vi "Methods to Tree Arr_2.vi"(7 "Action":T1, 10 "Class":string, 11 "Methods[]":T3(array[cluster])) -> (3 "Properties for Tree Out":T2(array[cluster]))   [LabVIEW 2023] (continued)
Tag", "Long name (localized)"="Tag:Delete"}, "Method Flags"={"IsDeprecated"=FALSE, "IsPrivate"=FALSE, "IsScripting"=FALSE, "IsNotInRun-Time"=TRUE}, "Divider"=FALSE}, {"Class Info"={"Unique ID string"="74", "Parent ID string"="", "Class Name (unlocalized)"="ProjectItem", "Class Name (localized)"="ProjectItem"}, "Method Info"={"Unique ID string"="35b5380f", "Data name"="Get Tag Names", "Short name (localized)"="Get Tag Names", "Long name (localized)"="Tag:Get Names"}, "Method Flags"={"IsDeprecated"=FALSE, "IsPrivate"=FALSE, "IsScripting"=FALSE, "IsNotInRun-Time"=FALSE}, "Divider"=FALSE}, {"Class Info"={"Unique ID string"="74", "Parent ID string"="", "Class Name (unlocalized)"="ProjectItem", "Class Name (localized)"="ProjectItem"}, "Method Info"={"Unique ID string"="35b53810", "Data name"="Get All Descendents", "Short name (localized)"="Get All Descendents", "Long name (localized)"="Get All Descendents"}, "Method Flags"={"IsDeprecated"=FALSE, "IsPrivate"=FALSE, "IsScripting"=FALSE, "IsNotInRun-Time"=FALSE}, "Divider"=FALSE}, {"Class Info"={"Unique ID string"="74", "Parent ID string"="", "Class Name (unlocalized)"="ProjectItem", "Class Name (localized)"="ProjectItem"}, "Method Info"={"Unique ID string"="35b53811", "Data name"="Make Item Visible in Tree", "Short name (localized)"="Make Item Visible in Tree", "Long name (localized)"="Make Item Visible in Tree"}, "Method Flags"={"IsDeprecated"=FALSE, "IsPrivate"=TRUE, "IsScripting"=FALSE, "IsNotInRun-Time"=TRUE}, "Divider"=FALSE}, {"Class Info"={"Unique ID string"="74", "Parent ID string"="", "Class Name (unlocalized)"="ProjectItem", "Class Name (localized)"="ProjectItem"}, "Method Info"={"Unique ID string"="35b53812", "Data name"="SelectItem", "Short name (localized)"="SelectItem", "Long name (localized)"="Select Item"}, "Method Flags"={"IsDeprecated"=FALSE, "IsPrivate"=TRUE, "IsScripting"=FALSE, "IsNotInRun-Time"=TRUE}, "Divider"=FALSE}, {"Class Info"={"Unique ID string"="74", "Parent ID string"="", "Class Name (unlocalized)"="ProjectItem", "Class Name (localized)"="ProjectItem"}, "Method Info"={"Unique ID string"="35b53813", "Data name"="SimulateDragSelection", "Short name (localized)"="SimulateDragSelection", "Long name (localized)"="Simulate:Drag Selection"}, "Method Flags"={"IsDeprecated"=FALSE, "IsPrivate"=TRUE, "IsScripting"=FALSE, "IsNotInRun-Time"=TRUE}, "Divider"=FALSE}, {"Class Info"={"Unique ID string"="74", "Parent ID string"="", "Class Name (unlocalized)"="ProjectItem", "Class Name (localized)"="ProjectItem"}, "Method Info"={"Unique ID string"="35b53814", "Data name"="Simulate Copy", "Short name (localized)"="Simulate Copy", "Long name (localized)"="Simulate:Copy"}, "Method Flags"={"IsDeprecated"=FALSE, "IsPrivate"=TRUE, "IsScripting"=FALSE, "IsNotInRun-Time"=TRUE}, "Divider"=FALSE}, {"Class Info"={"Unique ID string"="74", "Parent ID string"="", "Class Name (unlocalized)"="ProjectItem", "Class Name (localized)"="ProjectItem"}, "Method Info"={"Unique ID string"="35b53815", "Data name"="Simulate Paste", "Short name (localized)"="Simulate Paste", "Long name (localized)"="Simulate:Paste"}, "Method Flags"={"IsDeprecated"=FALSE, "IsPrivate"=TRUE, "IsScripting"=FALSE, "IsNotInRun-Time"=TRUE}, "Divider"=FALSE}, {"Class Info"={"Unique ID string"="74", "Parent ID string"="", "Class Name (unlocalized)"="ProjectItem", "Class Name (localized)"="ProjectItem"}, "Method Info"={"Unique ID string"="35b53816", "Data name"="Simulate Drag To VI", "Short name (localized)"="Simulate Drag To VI", "Long name (localized)"="Simulate:Drag To VI"}, "Method Flags"={"IsDeprecated"=FALSE, "IsPrivate"=TRUE, "IsScripting"=FALSE, "IsNotInRun-Time"=TRUE}, "Divider"=FALSE}, {"Class Info"={"Unique ID string"="74", "Parent ID string"="", "Class Name (unlocalized)"="ProjectItem", "Class Name (localized)"="ProjectItem"}, "Method Info"={"Unique ID string"="35b53817", "Data name"="Simulate Paste To VI", "Short name (localized)"="Simulate Paste To VI", "Long name (localized)"="Simulate:Paste To VI"}, "Method Flags"={"IsDeprecated"=FALSE, "IsPrivate"=TRUE, "IsScripting"=FALSE, "IsNotInRun-Time"=TRUE}, "Divider"=FALSE}, {"Class Info"={"Unique ID string"="74", "Parent ID string"="", "Class Name (unlocalized)"="ProjectItem", "Class Name (localized)"="ProjectItem"}, "Method Info"={"Unique ID string"="35b53818", "Data name"="Simulate Drag From Paths", "Short name (localized)"="Simulate Drag From Paths", "Long name (localized)"="Simulate:Drag From Paths"}, "Method Flags"={"IsDeprecated"=FALSE, "IsPrivate"=TRUE, "IsScripting"=FALSE, "IsNotInRun-Time"=TRUE}, "Divider"=FALSE}, {"Class Info"={"Unique ID string"="74", "Parent ID string"="", "Class Name (unlocalized)"="ProjectItem", "Class Name (localized)"="ProjectItem"}, "Method Info"={"Unique ID string"="35b53819", "Data name"="Collapse", "Short name (localized)"="Collapse", "Long name (localized)"="Collapse"}, "Method Flags"={"IsDeprecated"=FALSE, "IsPrivate"=FALSE, "IsScripting"=FALSE, "IsNotInRun-Time"=TRUE}, "Divider"=FALSE}, {"Class Info"={"Unique ID string"="74", "Parent ID string"="", "Class Name (unlocalized)"="ProjectItem", "Class Name (localized)"="ProjectItem"}, "Method Info"={"Unique ID string"="35b5381a", "Data name"="Rename", "Short name (localized)"="Rename", "Long name (localized)"="Rename"}, "Method Flags"={"IsDeprecated"=FALSE, "IsPrivate"=TRUE, "IsScripting"=FALSE, "IsNotInRun-Time"=TRUE}, "Divider"=FALSE}, {"Class Info"={"Unique ID string"="74", "Parent ID string"="", "Class Name (unlocalized)"="ProjectItem", "Class Name (localized)"="ProjectItem"}, "Method Info"={"Unique ID string"="35b5381b", "Data name"="New from Template", "Short name (localized)"="New from Template", "Long name (localized)"="New from Template"}, "Method Flags"={"IsDeprecated"=FALSE, "IsPrivate"=TRUE, "IsScripting"=FALSE, "IsNotInRun-Time"=TRUE}, "Divider"=FALSE}, {"Class Info"={"Unique ID string"="74", "Parent ID string"="", "Class Name (unlocalized)"="ProjectItem", "Class Name (localized)"="ProjectItem"}, "Method Info"={"Unique ID string"="35b5381c", "Data name"="Suppress Project Dlgs", "Short name (localized)"="Suppress Project Dlgs", "Long name (localized)"="Suppress Project Dialogs"}, "Method Flags"={"IsDeprecated"=FALSE, "IsPrivate"=TRUE, "IsScripting"=FALSE, "IsNotInRun-Time"=TRUE}, "Divider"=FALSE}, {"Class Info"={"Unique ID string"="74", "Parent ID string"="", "Class Name (unlocalized)"="ProjectItem", "Class Name (localized)"="ProjectItem"}, "Method Info"={"Unique ID string"="35b5381d", "Data name"="SimulateNotify", "Short name (localized)"="SimulateNotify", "Long name (localized)"="Simulate:Notify"}, "Method Flags"={"IsDeprecated"=FALSE, "IsPrivate"=TRUE, "IsScripting"=FALSE, "IsNotInRun-Time"=TRUE}, "Divider"=FALSE}, {"Class Info"={"Unique ID string"="74", "Parent ID string"="", "Class Name (unlocalized)"="ProjectItem", "Class Name (localized)"="ProjectItem"}, "Method Info"={"Unique ID string"="35b5381e", "Data name"="SCC Get Info", "Short name (localized)"="SCC Get Info", "Long name (localized)"="SCC Get Info"}, "Method Flags"={"IsDeprecated"=FALSE, "IsPrivate"=TRUE, "IsScripting"=FALSE, "IsNotInRun-Time"=TRUE}, "Divider"=FALSE}, {"Class Info"={"Unique ID string"="74", "Parent ID string"="", "Class Name (unlocalized)"="ProjectItem", "Class Name (localized)"="ProjectItem"}, "Method Info"={"Unique ID string"="35b5381f", "Data name"="Query Behavior", "Short name (localized)"="Query Behavior", "Long name (localized)"="Query Behavior"}, "Method Flags"={"IsDeprecated"=FALSE, "IsPrivate"=TRUE, "IsScripting"=FALSE, "IsNotInRun-Time"=TRUE}, "Divider"=FALSE}, {"Class Info"={"Unique ID string"="74", "Parent ID string"="", "Class Name (unlocalized)"="ProjectItem", "Class Name (localized)"="ProjectItem"}, "Method Info"={"Unique ID string"="35b53820", "Data name"="Move", "Short name (localized)"="Move", "Long name (localized)"="Move"}, "Method Flags"={"IsDeprecated"=FALSE, "IsPrivate"=TRUE, "IsScripting"=FALSE, "IsNotInRun-Time"=TRUE}, "Divider"=FALSE}, {"Class Info"={"Unique ID string"="74", "Parent ID string"="", "Class Name (unlocalized)"="ProjectItem", "Class Name (localized)"="ProjectItem"}, "Method Info"={"Unique ID string"="35b53821", "Data name"="Delete Privately", "Short name (localized)"="Delete Privately", "Long name (localized)"="Delete Privately (tell no outsiders)"}, "Method Flags"={"IsDeprecated"=FALSE, "IsPrivate"=TRUE, "IsScripting"=FALSE, "IsNotInRun-Time"=TRUE}, "Divider"=FALSE}, {"Class Info"={"Unique ID string"="74", "Parent ID string"="", "Class Name (unlocalized)"="ProjectItem", "Class Name (localized)"="ProjectItem"}, "Method Info"={"Unique ID string"="35b53822", "Data name"="Get XML Tag", "Short name (localized)"="Get XML Tag", "Long name (localized)"="Tag:Get XML Tag"}, "Method Flags"={"IsDeprecated"=FALSE, "IsPrivate"=FALSE, "IsScripting"=FALSE, "IsNotInRun-Time"=FALSE}, "Divider"=FALSE}, {"Class Info"={"Unique ID string"="74", "Parent ID string"="", "Class Name (unlocalized)"="ProjectItem", "Class Name (localized)"="ProjectItem"}, "Method Info"={"Unique ID string"="35b53823", "Data name"="Set XML Tag", "Short name (localized)"="Set XML Tag", "Long name (localized)"="Tag:Set XML Tag"}, "Method Flags"={"IsDeprecated"=FALSE, "IsPrivate"=FALSE, "IsScripting"=FALSE, "IsNotInRun-Time"=TRUE}, "Divider"=FALSE}, {"Class Info"={"Unique ID string"="74", "Parent ID string"="", "Class Name (unlocalized)"="ProjectItem", "Class Name (localized)"="ProjectItem"}, "Method Info"={"Unique ID string"="35b53824", "Data name"="AddItemFromMemory", "Short name (localized)"="AddItemFromMemory", "Long name (localized)"="Add Item From Memory"}, "Method Flags"={"IsDeprecated"=FALSE, "IsPrivate"=FALSE, "IsScripting"=FALSE, "IsNotInRun-Time"=TRUE}, "Divider"=FALSE}, {"Class Info"={"Unique ID string"="74", "Parent ID string"="", "Class Name (unlocalized)"="ProjectItem", "Class Name (localized)"="ProjectItem"}, "Method Info"={"Unique ID string"="35b53825", "Data name"="NotifyItemChanged", "Short name (localized)"="NotifyItemChanged", "Long name (localized)"="Notify Item Changed"}, "Method Flags"={"IsDeprecated"=FALSE, "IsPrivate"=TRUE, "IsScripting"=FALSE, "IsNotInRun-Time"=TRUE}, "Divider"=FALSE}, {"Class Info"={"Unique ID string"="74", "Parent ID string"="", "Class Name (unlocalized)"="ProjectItem", "Class Name (localized)"="ProjectItem"}, "Method Info"={"Unique ID string"="35b53826", "Data name"="Expand", "Short name (localized)"="Expand", "Long name (localized)"="Expand"}, "Method Flags"={"IsDeprecated"=FALSE, "IsPrivate"=FALSE, "IsScripting"=FALSE, "IsNotInRun-Time"=TRUE}, "Divider"=FALSE}, {"Class Info"={"Unique ID string"="74", "Parent ID string"="", "Class Name (unlocalized)"="ProjectItem", "Class Name (localized)"="ProjectItem"}, "Method Info"={"Unique ID string"="35b53827", "Data name"="Arrange By", "Short name (localized)"="Arrange By", "Long name (localized)"="Arrange By"}, "Method Flags"={"IsDeprecated"=FALSE, "IsPrivate"=TRUE, "IsScripting"=FALSE, "IsNotInRun-Time"=TRUE}, "Divider"=FALSE}, {"Class Info"={"Unique ID string"="74", "Parent ID string"="", "Class Name (unlocalized)"="ProjectItem", "Class Name (localized)"="ProjectItem"}, "Method Info"={"Unique ID string"="35b53828", "Data name"="SetUrl", "Short name (localized)"="SetUrl", "Long name (localized)"="Set Url"}, "Method Flags"={"IsDeprecated"=FALSE, "IsPrivate"=TRUE, "IsScripting"=FALSE, "IsNotInRun-Time"=TRUE}, "Divider"=FALSE}, {"Class Info"={"Unique ID string"="74", "Parent ID string"="", "Class Name (unlocalized)"="ProjectItem", "Class Name (localized)"="ProjectItem"}, "Method Info"={"Unique ID string"="35b53829", "Data name"="Get All Descendents2", "Short name (localized)"="Get All Descendents2", "Long name (localized)"="Get All Descendents2"}, "Method Flags"={"IsDeprecated"=FALSE, "IsPrivate"=TRUE, "IsScripting"=FALSE, "IsNotInRun-Time"=FALSE}, "Divider"=FALSE}, {"Class Info"={"Unique ID string"="74", "Parent ID string"="", "Class Name (unlocalized)"="ProjectItem", "Class Name (localized)"="ProjectItem"}, "Method Info"={"Unique ID string"="35b5382a", "Data name"="GetFindResults", "Short name (localized)"="GetFindResults", "Long name (localized)"="GetFindResults"}, "Method Flags"={"IsDeprecated"=FALSE, "IsPrivate"=TRUE, "IsScripting"=FALSE, "IsNotInRun-Time"=FALSE}, "Divider"=FALSE}, {"Class Info"={"Unique ID string"="74", "Parent ID string"="", "Class Name (unlocalized)"="ProjectItem", "Class Name (localized)"="ProjectItem"}, "Method Info"={"Unique ID string"="35b5382b", "Data name"="Convert to Auto-populating Folder", "Short name (localized)"="Convert to Auto-populating Folder", "Long name (localized)"="Convert to Auto-populating Folder"}, "Method Flags"={"IsDeprecated"=FALSE, "IsPrivate"=FALSE, "IsScripting"=FALSE, "IsNotInRun-Time"=TRUE}, "Divider"=FALSE}, {"Class Info"={"Unique ID string"="74", "Parent ID string"="", "Class Name (unlocalized)"="ProjectItem", "Class Name (localized)"="ProjectItem"}, "Method Info"={"Unique ID string"="35b5382c", "Data name"="Stop Auto-populating", "Short name (localized)"="Stop Auto-populating", "Long name (localized)"="Stop Auto-populating"}, "Method Flags"={"IsDeprecated"=FALSE, "IsPrivate"=FALSE, "IsScripting"=FALSE, "IsNotInRun-Time"=TRUE}, "Divider"=FALSE}, {"Class Info"={"Unique ID string"="74", "Parent ID string"="", "Class Name (unlocalized)"="ProjectItem", "Class Name (localized)"="ProjectItem"}, "Method Info"={"Unique ID string"="35b5382d", "Data name"="Delete On Disk", "Short name (localized)"="Delete On Disk", "Long name (localized)"="Delete On Disk"}, "Method Flags"={"IsDeprecated"=FALSE, "IsPrivate"=TRUE, "IsScripting"=FALSE, "IsNotInRun-Time"=FALSE}, "Divider"=FALSE}, {"Class Info"={"Unique ID string"="74", "Parent ID string"="", "Class Name (unlocalized)"="ProjectItem", "Class Name (localized)"="ProjectItem"}, "Method Info"={"Unique ID string"="35b5382e", "Data name"="ListOfReferProjItems", "Short name (localized)"="ListOfReferProjItems", "Long name (localized)"="List of Refer ProjectItems"}, "Method Flags"={"IsDeprecated"=FALSE, "IsPrivate"=TRUE, "IsScripting"=FALSE, "IsNotInRun-Time"=FALSE}, "Divider"=FALSE}, {"Class Info"={"Unique ID string"="74", "Parent ID string"="", "Class Name (unlocalized)"="ProjectItem", "Class Name (localized)"="ProjectItem"}, "Method Info"={"Unique ID string"="35b5382f", "Data name"="ReplaceWithProjItem", "Short name (localized)"="ReplaceWithProjItem", "Long name (localized)"="Replace With Item in Project"}, "Method Flags"={"IsDeprecated"=FALSE, "IsPrivate"=TRUE, "IsScripting"=FALSE, "IsNotInRun-Time"=FALSE}, "Divider"=FALSE}, {"Class Info"={"Unique ID string"="74", "Parent ID string"="", "Class Name (unlocalized)"="ProjectItem", "Class Name (localized)"="ProjectItem"}, "Method Info"={"Unique ID string"="35b53830", "Data name"="Choose Substitute", "Short name (localized)"="Choose Substitute", "Long name (localized)"="Choose Substitute"}, "Method Flags"={"IsDeprecated"=FALSE, "IsPrivate"=TRUE, "IsScripting"=FALSE, "IsNotInRun-Time"=FALSE}, "Divider"=FALSE}, {"Class Info"={"Unique ID string"="74", "Parent ID string"="", "Class Name (unlocalized)"="ProjectItem", "Class Name (localized)"="ProjectItem"}, "Method Info"={"Unique ID string"="35b53831", "Data name"="AddMultipleItems", "Short name (localized)"="AddMultipleItems", "Long name (localized)"="AddMultipleItems"}, "Method Flags"={"IsDeprecated"=FALSE, "IsPrivate"=TRUE, "IsScripting"=FALSE, "IsNotInRun-Time"=FALSE}, "Divider"=FALSE}, {"Class Info"={"Unique ID string"="74", "Parent ID string"="", "Class Name (unlocalized)"="ProjectItem", "Class Name (localized)"="ProjectItem"}, "Method Info"={"Unique ID string"="35b53832", "Data name"="ForceDelete", "Short name (localized)"="ForceDelete", "Long name (localized)"="ForceDelete"}, "Method Flags"={"IsDeprecated"=FALSE, "IsPrivate"=TRUE, "IsScripting"=FALSE, "IsNotInRun-Time"=FALSE}, "Divider"=FALSE}, {"Class Info"={"Unique ID string"="74", "Parent ID string"="", "Class Name (unlocalized)"="ProjectItem", "Class Name (localized)"="ProjectItem"}, "Method Info"={"Unique ID string"="35b53833", "Data name"="Bounds", "Short name (localized)"="Bounds", "Long name (localized)"="Bounds"}, "Method Flags"={"IsDeprecated"=FALSE, "IsPrivate"=TRUE, "IsScripting"=FALSE, "IsNotInRun-Time"=FALSE}, "Divider"=FALSE}, {"Class Info"={"Unique ID string"="74", "Parent ID string"="", "Class Name (unlocalized)"="ProjectItem", "Class Name (localized)"="ProjectItem"}, "Method Info"={"Unique ID string"="35b53834", "Data name"="GetVariableURLs", "Short name (localized)"="GetVariableURLs", "Long name (localized)"="Get Variable URLs"}, "Method Flags"={"IsDeprecated"=FALSE, "IsPrivate"=TRUE, "IsScripting"=FALSE, "IsNotInRun-Time"=TRUE}, "Divider"=FALSE}, {"Class Info"={"Unique ID string"="74", "Parent ID string"="", "Class Name (unlocalized)"="ProjectItem", "Class Name (localized)"="ProjectItem"}, "Method Info"={"Unique ID string"="35b53835", "Data name"="AddItemFromMemoryPrivately", "Short name (localized)"="AddItemFromMemoryPrivately", "Long name (localized)"="Add Item From Memory Privately"}, "Method Flags"={"IsDeprecated"=FALSE, "IsPrivate"=TRUE, "IsScripting"=FALSE, "IsNotInRun-Time"=TRUE}, "Divider"=FALSE}, {"Class Info"={"Unique ID string"="74", "Parent ID string"="", "Class Name (unlocalized)"="ProjectItem", "Class Name (localized)"="ProjectItem"}, "Method Info"={"Unique ID string"="35b53836", "Data name"="Get Library Access Scope", "Short name (localized)"="Get Library Access Scope", "Long name (localized)"="Get Library Access Scope"}, "Method Flags"={"IsDeprecated"=FALSE, "IsPrivate"=TRUE, "IsScripting"=FALSE, "IsNotInRun-Time"=TRUE}, "Divider"=FALSE}, {"Class Info"={"Unique ID string"="74", "Parent ID string"="", "Class Name (unlocalized)"="ProjectItem", "Class Name (localized)"="ProjectItem"}, "Method Info"={"Unique ID string"="35b53837", "Data name"="Replace Item With", "Short name (localized)"="Replace Item With", "Long name (localized)"="Replace Item With"}, "Method Flags"={"IsDeprecated"=FALSE, "IsPrivate"=FALSE, "IsScripting"=FALSE, "IsNotInRun-Time"=TRUE}, "Divider"=FALSE}, {"Class Info"={"Unique ID string"="75", "Parent ID string"="36", "Class Name (unlocalized)"="Pane", "Class Name (localized)"="Pane"}, "Method Info"={"Unique ID string"="64afa400", "Data name"="MakeSpace", "Short name (localized)"="MakeSpace", "Long name (localized)"="Make Space"}, "Method Flags"={"IsDeprecated"=FALSE, "IsPrivate"=FALSE, "IsScripting"=TRUE, "IsNotInRun-Time"=TRUE}, "Divider"=FALSE}, {"Class Info"={"Unique ID string"="75", "Parent ID string"="36", "Class Name (unlocalized)"="Pane", "Class Name (localized)"="Pane"}, "Method Info"={"Unique ID string"="64afa402", "Data name"="Select All", "Short name (localized)"="Select All", "Long name (localized)"="Select All"}, "Method Flags"={"IsDeprecated"=FALSE, "IsPrivate"=FALSE, "IsScripting"=TRUE, "IsNotInRun-Time"=TRUE}, "Divider"=FALSE}, {"Class Info"={"Unique ID string"="75", "Parent ID string"="36", "Class Name (unlocalized)"="Pane", "Class Name (localized)"="Pane"}, "Method Info"={"Unique ID string"="64afa403", "Data name"="Paste Selection", "Short name (localized)"="Paste Selection", "Long name (localized)"="Paste Selection"}, "Method Flags"={"IsDeprecated"=FALSE, "IsPrivate"=FALSE, "IsScripting"=TRUE, "IsNotInRun-Time"=TRUE}, "Divider"=FALSE}, {"Class Info"={"Unique ID string"="75", "Parent ID string"="36", "Class Name (unlocalized)"="Pane", "Class Name (localized)"="Pane"}, "Method Info"={"Unique ID string"="64afa404", "Data name"="Group Objects", "Short name (localized)"="Group Objects", "Long name (localized)"="Group Objects"}, "Method Flags"={"IsDeprecated"=FALSE, "IsPrivate"=FALSE, "IsScripting"=TRUE, "IsNotInRun-Time"=TRUE}, "Divider"=FALSE}, {"Class Info"={"Unique ID string"="75", "Parent ID string"="36", "Class Name (unlocalized)"="Pane", "Class Name (localized)"="Pane"}, "Method Info"={"Unique ID string"="64afa405", "Data name"="Lock Objects", "Short name (localized)"="Lock Objects", "Long name (localized)"="Lock Objects"}, "Method Flags"={"IsDeprecated"=FALSE, "IsPrivate"=FALSE, "IsScripting"=TRUE, "IsNotInRun-Time"=TRUE}, "Divider"=FALSE}, {"Class Info"={"Unique ID string"="75", "Parent ID string"="36", "Class Name (unlocalized)"="Pane", "Class Name (localized)"="Pane"}, "Method Info"={"Unique ID string"="64afa406", "Data name"="Ungroup Objects", "Short name (localized)"="Ungroup Objects", "Long name (localized)"="Ungroup Objects"}, "Method Flags"={"IsDeprecated"=FALSE, "IsPrivate"=FALSE, "IsScripting"=TRUE, "IsNotInRun-Time"=TRUE}, "Divider"=FALSE}, {"Class Info"={"Unique ID string"="75", "Parent ID string"="36", "Class Name (unlocalized)"="Pane", "Class Name (localized)"="Pane"}, "Method Info"={"Unique ID string"="64afa407", "Data name"="Unlock Objects", "Short name (localized)"="Unlock Objects", "Long name (localized)"="Unlock Objects"}, "Method Flags"={"IsDeprecated"=FALSE, "IsPrivate"=FALSE, "IsScripting"=TRUE, "IsNotInRun-Time"=TRUE}, "Divider"=FALSE}, {"Class Info"={"Unique ID string"="75", "Parent ID string"="36", "Class Name (unlocalized)"="Pane", "Class Name (localized)"="Pane"}, "Method Info"={"Unique ID string"="64afa408", "Data name"="Set Scaling", "Short name (localized)"="Set Scaling", "Long name (localized)"="Set Scaling Mode"}, "Method Flags"={"IsDeprecated"=FALSE, "IsPrivate"=FALSE, "IsScripting"=FALSE, "IsNotInRun-Time"=FALSE}, "Divider"=FALSE}, {"Class Info"={"Unique ID string"="75", "Parent ID string"="36", "Class Name (unlocalized)"="Pane", "Class Name (localized)"="Pane"}, "Method Info"={"Unique ID string"="64afa409", "Data name"="Get Scaling", "Short name (localized)"="Get Scaling", "Long name (localized)"="Get Scaling Mode"}, "Method Flags"={"IsDeprecated"=FALSE, "IsPrivate"=FALSE, "IsScripting"=FALSE, "IsNotInRun-Time"=FALSE}, "Divider"=FALSE}, {"Class Info"={"Unique ID string"="75", "Parent ID string"="36", "Class Name (unlocalized)"="Pane", "Class Name (localized)"="Pane"}, "Method Info"={"Unique ID string"="64afa40a", "Data name"="CvtPaneToPanelCoords", "Short name (localized)"="CvtPaneToPanelCoords", "Long name (localized)"="Convert Pane To Panel Coordinates"}, "Method Flags"={"IsDeprecated"=FALSE, "IsPrivate"=FALSE, "IsScripting"=FALSE, "IsNotInRun-Time"=FALSE}, "Divider"=FALSE}, {"Class Info"={"Unique ID string"="75", "Parent ID string"="36", "Class Name (unlocalized)"="Pane", "Class Name (localized)"="Pane"}, "Method Info"={"Unique ID string"="64afa40b", "Data name"="CvtPanelToPaneCoords", "Short name (localized)"="CvtPanelToPaneCoords", "Long name (localized)"="Convert Panel To Pane Coordinates"}, "Method Flags"={"IsDeprecated"=FALSE, "IsPrivate"=FALSE, "IsScripting"=FALSE, "IsNotInRun-Time"=FALSE}, "Divider"=FALSE}, {"Class Info"={"Unique ID string"="80", "Parent ID string"="74", "Class Name (unlocalized)"="Library", "Class Name (localized)"="Library"}, "Method Info"={"Unique ID string"="4d10e400", "Data name"="Set Source Scope", "Short name (localized)"="Set Source Scope", "Long name (localized)"="Source Scope:Set"}, "Method Flags"={"IsDeprecated"=FALSE, "IsPrivate"=FALSE, "IsScripting"=FALSE, "IsNotInRun-Time"=TRUE}, "Divider"=FALSE}, {"Class Info"={"Unique ID string"="80", "Parent ID string"="74", "Class Name (unlocalized)"="Library", "Class Name (localized)"="Library"}, "Method Info"={"Unique ID string"="4d10e401", "Data name"="Get Source Scope", "Short name (localized)"="Get Source Scope", "Long name (localized)"="Source Scope:Get"}, "Method Flags"={"IsDeprecated"=FALSE, "IsPrivate"=FALSE, "IsScripting"=FALSE, "IsNotInRun-Time"=FALSE}, "Divider"=FALSE}, {"Class Info"={"Unique ID string"="80", "Parent ID string"="74", "Class Name (unlocalized)"="Library", "Class Name (localized)"="Library"}, "Method Info"={"Unique ID string"="4d10e402", "Data name"="Set Lock State", "Short name (localized)"="Set Lock State", "Long name (localized)"="Lock State:Set"}, "Method Flags"={"IsDeprecated"=FALSE, "IsPrivate"=FALSE, "IsScripting"=FALSE, "IsNotInRun-Time"=TRUE}, "Divider"=FALSE}, {"Class Info"={"Unique ID string"="80", "Parent ID string"="74", "Class Name (unlocalized)"="Library", "Class Name (localized)"="Library"}, "Method Info"={"Unique ID string"="4d10e403", "Data name"="Get Lock State", "Short name (localized)"="Get Lock State", "Long name (localized)"="Lock State:Get"}, "Method Flags"={"IsDeprecated"=FALSE, "IsPrivate"=FALSE, "IsScripting"=FALSE, "IsNotInRun-Time"=FALSE}, "Divider"=FALSE}, {"Class Info"={"Unique ID string"="80", "Parent ID string"="74", "Class Name (unlocalized)"="Library", "Class Name (localized)"="Library"}, "Method Info"={"Unique ID string"="4d10e404", "Data name"="Get Lib Tag", "Short name (localized)"="Get Lib Tag", "Long name (localized)"="Library Tag:Get"}, "Method Flags"={"IsDeprecated"=FALSE, "IsPrivate"=FALSE, "IsScripting"=FALSE, "IsNotInRun-Time"=FALSE}, "Divider"=FALSE}, {"Class Info"={"Unique ID string"="80", "Parent ID string"="74", "Class Name (unlocalized)"="Library", "Class Name (localized)"="Library"}, "Method Info"={"Unique ID string"="4d10e405", "Data name"="Set Lib Tag", "Short name (localized)"="Set Lib Tag", "Long name (localized)"="Library Tag:Set"}, "Method Flags"={"IsDeprecated"=FALSE, "IsPrivate"=FALSE, "IsScripting"=FALSE, "IsNotInRun-Time"=TRUE}, "Divider"=FALSE}, {"Class Info"={"Unique ID string"="80", "Parent ID string"="74", "Class Name (unlocalized)"="Library", "Class Name (localized)"="Library"}, "Method Info"={"Unique ID string"="4d10e406", "Data name"="Delete Lib Tag", "Short name (localized)"="Delete Lib Tag", "Long name (localized)"="Library Tag:Delete"}, "Method Flags"={"IsDeprecated"=FALSE, "IsPrivate"=FALSE, "IsScripting"=FALSE, "IsNotInRun-Time"=TRUE}, "Divider"=FALSE}, {"Class Info"={"Unique ID string"="80", "Parent ID string"="74", "Class Name (unlocalized)"="Library", "Class Name (localized)"="Library"}, "Method Info"={"Unique ID string"="4d10e407", "Data name"="Get Lib Tag Names", "Short name (localized)"="Get Lib Tag Names", "Long name (localized)"="Library Tag:Get Names"}, "Method Flags"={"IsDeprecated"=FALSE, "IsPrivate"=FALSE, "IsScripting"=FALSE, "IsNotInRun-Time"=FALSE}, "Divider"=FALSE}, {"Class Info"={"Unique ID string"="80", "Parent ID string"="74", "Class Name (unlocalized)"="Library", "Class Name (localized)"="Library"}, "Method Info"={"Unique ID string"="4d10e408", "Data name"="Save", "Short name (localized)"="Save", "Long name (localized)"="Save:Library"}, "Method Flags"={"IsDeprecated"=FALSE, "IsPrivate"=FALSE, "IsScripting"=FALSE, "IsNotInRun-Time"=TRUE}, "Divider"=FALSE}, {"Class Info"={"Unique ID string"="80", "Parent ID string"="74", "Class Name (unlocalized)"="Library", "Class Name (localized)"="Library"}, "Method Info"={"Unique ID string"="4d10e409", "Data name"="Get Icon", "Short name (localized)"="Get Icon", "Long name (localized)"="Icon:Get"}, "Method Flags"={"IsDeprecated"=FALSE, "IsPrivate"=FALSE, "IsScripting"=FALSE, "IsNotInRun-Time"=FALSE}, "Divider"=FALSE}, {"Class Info"={"Unique ID string"="80", "Parent ID string"="74", "Class Name (unlocalized)"="Library", "Class Name (localized)"="Library"}, "Method Info"={"Unique ID string"="4d10e40a", "Data name"="Set Icon", "Short name (localized)"="Set Icon", "Long name (localized)"="Icon:Set"}, "Method Flags"={"IsDeprecated"=FALSE, "IsPrivate"=FALSE, "IsScripting"=FALSE, "IsNotInRun-Time"=TRUE}, "Divider"=FALSE}, {"Class Info"={"Unique ID string"="80", "Parent ID string"="74", "Class Name (unlocalized)"="Library", "Class Name (localized)"="Library"}, "Method Info"={"Unique ID string"="4d10e40b", "Data name"="Debug Apply From Other Context", "Short name (localized)"="Debug Apply From Other Context", "Long name (localized)"="Debug Apply From Other Context"}, "Method Flags"={"IsDeprecated"=FALSE, "IsPrivate"=TRUE, "IsScripting"=FALSE, "IsNotInRun-Time"=TRUE}, "Divider"=FALSE}, {"Class Info"={"Unique ID string"="80", "Parent ID string"="74", "Class Name (unlocalized)"="Library", "Class Name (localized)"="Library"}, "Method Info"={"Unique ID string"="4d10e40c", "Data name"="Revert", "Short name (localized)"="Revert", "Long name (localized)"="Revert"}, "Method Flags"={"IsDeprecated"=FALSE, "IsPrivate"=TRUE, "IsScripting"=FALSE, "IsNotInRun-Time"=TRUE}, "Divider"=FALSE}, {"Class Info"={"Unique ID string"="80", "Parent ID string"="74", "Class Name (unlocalized)"="Library", "Class Name (localized)"="Library"}, "Method Info"={"Unique ID string"="4d10e40d", "Data name"="Synchronize In All Contexts", "Short name (localized)"="Synchronize In All Contexts", "Long name (localized)"="Synchronize In All Contexts"}, "Method Flags"={"IsDeprecated"=FALSE, "IsPrivate"=TRUE, "IsScripting"=FALSE, "IsNotInRun-Time"=TRUE}, "Divider"=FALSE}, {"Class Info"={"Unique ID string"="80", "Parent ID string"="74", "Class Name (unlocalized)"="Library", "Class Name (localized)"="Library"}, "Method Info"={"Unique ID string"="4d10e40e", "Data name"="Save a Copy", "Short name (localized)"="Save a Copy", "Long name (localized)"="Save:Copy"}, "Method Flags"={"IsDeprecated"=FALSE, "IsPrivate"=FALSE, "IsScripting"=FALSE, "IsNotInRun-Time"=TRUE}, "Divider"=FALSE}, {"Class Info"={"Unique ID string"="80", "Parent ID string"="74", "Class Name (unlocalized)"="Library", "Class Name (localized)"="Library"}, "Method Info"={"Unique ID string"="4d10e40f", "Data name"="Set Temp Lock State", "Short name (localized)"="Set Temp Lock State", "Long name (localized)"="Lock State:Set Temp Lock State"}, "Method Flags"={"IsDeprecated"=FALSE, "IsPrivate"=TRUE, "IsScripting"=FALSE, "IsNotInRun-Time"=TRUE}, "Divider"=FALSE}, {"Class Info"={"Unique ID string"="80", "Parent ID string"="74", "Class Name (unlocalized)"="Library", "Class Name (localized)"="Library"}, "Method Info"={"Unique ID string"="4d10e410", "Data name"="DisconnectFromLibrary", "Short name (localized)"="DisconnectFromLibrary", "Long name (localized)"="Disconnect From Library"}, "Method Flags"={"IsDeprecated"=FALSE, "IsPrivate"=FALSE, "IsScripting"=FALSE, "IsNotInRun-Time"=TRUE}, "Divider"=FALSE}, {"Class Info"={"Unique ID string"="80", "Parent ID string"="74", "Class Name (unlocalized)"="Library", "Class Name (localized)"="Library"}, "Method Info"={"Unique ID string"="4d10e411", "Data name"="Save For Previous", "Short name (localized)"="Save For Previous", "Long name (localized)"="Save:For Previous"}, "Method Flags"={"IsDeprecated"=FALSE, "IsPrivate"=FALSE, "IsScripting"=FALSE, "IsNotInRun-Time"=TRUE}, "Divider"=FALSE}, {"Class Info"={"Unique ID string"="80", "Parent ID string"="74", "Class Name (unlocalized)"="Library", "Class Name (localized)"="Library"}, "Method Info"={"Unique ID string"="4d10e412", "Data name"="LibraryData.Add", "Short name (localized)"="LibraryData.Add", "Long name (localized)"="Library Data:Add"}, "Method Flags"={"IsDeprecated"=FALSE, "IsPrivate"=TRUE, "IsScripting"=FALSE, "IsNotInRun-Time"=FALSE}, "Divider"=FALSE}, {"Class Info"={"Unique ID string"="80", "Parent ID string"="74", "Class Name (unlocalized)"="Library", "Class Name (localized)"="Library"}, "Method Info"={"Unique ID string"="4d10e413", "Data name"="LibraryData.Get", "Short name (localized)"="LibraryData.Get", "Long name (localized)"="Library Data:Get"}, "Method Flags"={"IsDeprecated"=FALSE, "IsPrivate"=TRUE, "IsScripting"=FALSE, "IsNotInRun-Time"=FALSE}, "Divider"=FALSE}, {"Class Info"={"Unique ID string"="80", "Parent ID string"="74", "Class Name (unlocalized)"="Library", "Class Name (localized)"="Library"}, "Method Info"={"Unique ID string"="4d10e414", "Data name"="Save to buffer", "Short name (localized)"="Save to buffer", "Long name (localized)"="Save:Save to Buffer"}, "Method Flags"={"IsDeprecated"=FALSE, "IsPrivate"=TRUE, "IsScripting"=FALSE, "IsNotInRun-Time"=FALSE}, "Divider"=FALSE}, {"Class Info"={"Unique ID string"="80", "Parent ID string"="74", "Class Name (unlocalized)"="Library", "Class Name (localized)"="Library"}, "Method Info"={"Unique ID string"="4d10e415", "Data name"="Set DocMod", "Short name (localized)"="Set DocMod", "Long name (localized)"="Set DocMod"}, "Method Flags"={"IsDeprecated"=FALSE, "IsPrivate"=TRUE, "IsScripting"=FALSE, "IsNotInRun-Time"=TRUE}, "Divider"=FALSE}, {"Class Info"={"Unique ID string"="80", "Parent ID string"="74", "Class Name (unlocalized)"="Library", "Class Name (localized)"="Library"}, "Method Info"={"Unique ID string"="4d10e416", "Data name"="ApplyIconToVIs", "Short name (localized)"="ApplyIconToVIs", "Long name (localized)"="Apply Icon To Existing VI Items"}, "Method Flags"={"IsDeprecated"=FALSE, "IsPrivate"=FALSE, "IsScripting"=FALSE, "IsNotInRun-Time"=TRUE}, "Divider"=FALSE}, {"Class Info"={"Unique ID string"="80", "Parent ID string"="74", "Class Name (unlocalized)"="Library", "Class Name (localized)"="Library"}, "Method Info"={"Unique ID string"="4d10e417", "Data name"="Save.Target Library", "Short name (localized)"="Save.Target Library", "Long name (localized)"="Save:Target Library"}, "Method Flags"={"IsDeprecated"=FALSE, "IsPrivate"=TRUE, "IsScripting"=FALSE, "IsNotInRun-Time"=TRUE}, "Divider"=FALSE}, {"Class Info"={"Unique ID string"="80", "Parent ID string"="74", "Class Name (unlocalized)"="Library", "Class Name (localized)"="Library"}, "Method Info"={"Unique ID string"="4d10e418", "Data name"="Amalgamation.SetEditsOnlyOnThis", "Short name (localized)"="Amalgamation.SetEditsOnlyOnThis", "Long name (localized)"="Amalgamation:Set Edits Only On This"}, "Method Flags"={"IsDeprecated"=FALSE, "IsPrivate"=TRUE, "IsScripting"=FALSE, "IsNotInRun-Time"=FALSE}, "Divider"=FALSE}, {"Class Info"={"Unique ID string"="80", "Parent ID string"="74", "Class Name (unlocalized)"="Library", "Class Name (localized)"="Library"}, "Method Info"={"Unique ID string"="4d10e419", "Data name"="HiliteInProjectWindow", "Short name (localized)"="HiliteInProjectWindow", "Long name (localized)"="Hilite In Project Window"}, "Method Flags"={"IsDeprecated"=FALSE, "IsPrivate"=FALSE, "IsScripting"=FALSE, "IsNotInRun-Time"=TRUE}, "Divider"=FALSE}, {"Class Info"={"Unique ID string"="80", "Parent ID string"="74", "Class Name (unlocalized)"="Library", "Class Name (localized)"="Library"}, "Method Info"={"Unique ID string"="4d10e41a", "Data name"="Amalgamation.ShouldDisposePieceOnNextSave", "Short name (localized)"="Amalgamation.ShouldDisposePieceOnNextSave", "Long name (localized)"="Amalgamation:ShouldDisposePieceOnNextSave"}, "Method Flags"={"IsDeprecated"=FALSE, "IsPrivate"=TRUE, "IsScripting"=FALSE, "IsNotInRun-Time"=FALSE}, "Divider"=FALSE}, {"Class Info"={"Unique ID string"="80", "Parent ID string"="74", "Class Name (unlocalized)"="Library", "Class Name (localized)"="Library"}, "Method Info"={"Unique ID string"="4d10e41b", "Data name"="AddFriendLibrary", "Short name (localized)"="AddFriendLibrary", "Long name (localized)"="Friends:Add Friend Library"}, "Method Flags"={"IsDeprecated"=FALSE, "IsPrivate"=FALSE, "IsScripting"=FALSE, "IsNotInRun-Time"=TRUE}, "Divider"=FALSE}, {"Class Info"={"Unique ID string"="80", "Parent ID string"="74", "Class Name (unlocalized)"="Library", "Class Name (localized)"="Library"}, "Method Info"={"Unique ID string"="4d10e41c", "Data name"="AddFriendVI", "Short name (localized)"="AddFriendVI", "Long name (localized)"="Friends:Add Friend VI"}, "Method Flags"={"IsDeprecated"=FALSE, "IsPrivate"=FALSE, "IsScripting"=FALSE, "IsNotInRun-Time"=TRUE}, "Divider"=FALSE}, {"Class Info"={"Unique ID string"="80", "Parent ID string"="74", "Class Name (unlocalized)"="Library", "Class Name (localized)"="Library"}, "Method Info"={"Unique ID string"="4d10e41d", "Data name"="RemoveFriend", "Short name (localized)"="RemoveFriend", "Long name (localized)"="Friends:Remove Friended VI or Library"}, "Method Flags"={"IsDeprecated"=FALSE, "IsPrivate"=FALSE, "IsScripting"=FALSE, "IsNotInRun-Time"=TRUE}, "Divider"=FALSE}, {"Class Info"={"Unique ID string"="80", "Parent ID string"="74", "Class Name (unlocalized)"="Library", "Class Name (localized)"="Library"}, "Method Info"={"Unique ID string"="4d10e41e", "Data name"="SetPath", "Short name (localized)"="SetPath", "Long name (localized)"="SetPath"}, "Method Flags"={"IsDeprecated"=FALSE, "IsPrivate"=TRUE, "IsScripting"=FALSE, "IsNotInRun-Time"=TRUE}, "Divider"=FALSE}, {"Class Info"={"Unique ID string"="80", "Parent ID string"="74", "Class Name (unlocalized)"="Library", "Class Name (localized)"="Library"}, "Method Info"={"Unique ID string"="4d10e41f", "Data name"="SetPathAsPacked", "Short name (localized)"="SetPathAsPacked", "Long name (localized)"="Set Path As Packed"}, "Method Flags"={"IsDeprecated"=FALSE, "IsPrivate"=TRUE, "IsScripting"=FALSE, "IsNotInRun-Time"=TRUE}, "Divider"=FALSE}, {"Class Info"={"Unique ID string"="80", "Parent ID string"="74", "Class Name (unlocalized)"="Library", "Class Name (localized)"="Library"}, "Method Info"={"Unique ID string"="4d10e420", "Data name"="DisconnectVariablesFromTypedefs", "Short name (localized)"="DisconnectVariablesFromTypedefs", "Long name (localized)"="Disconnect Variables From Typedefs"}, "Method Flags"={"IsDeprecated"=FALSE, "IsPrivate"=FALSE, "IsScripting"=FALSE, "IsNotInRun-Time"=FALSE}, "Divider"=FALSE}, {"Class Info"={"Unique ID string"="80", "Parent ID string"="74", "Class Name (unlocalized)"="Library", "Class Name (localized)"="Library"}, "Method Info"={"Unique ID string"="4d10e421", "Data name"="Set Source Scope And Propagate", "Short name (localized)"="Set Source Scope And Propagate", "Long name (localized)"="Source Scope:Set and Propagate"}, "Method Flags"={"IsDeprecated"=FALSE, "IsPrivate"=FALSE, "IsScripting"=FALSE, "IsNotInRun-Time"=TRUE}, "Divider"=FALSE}, {"Class Info"={"Unique ID string"="80", "Parent ID string"="74", "Class Name (unlocalized)"="Library", "Class Name (localized)"="Library"}, "Method Info"={"Unique ID string"="4d10e423", "Data name"="License.Get License Status", "Short name (localized)"="License.Get License Status", "Long name (localized)"="License:Get License Status"}, "Method Flags"={"IsDeprecated"=FALSE, "IsPrivate"=TRUE, "IsScripting"=FALSE, "IsNotInRun-Time"=FALSE}, "Divider"=FALSE}, {"Class Info"={"Unique ID string"="80", "Parent ID string"="74", "Class Name (unlocalized)"="Library", "Class Name (localized)"="Library"}, "Method Info"={"Unique ID string"="4d10e424", "Data name"="Packed Library.GetNonExportedPaths", "Short name (localized)"="Packed Library.GetNonExportedPaths", "Long name (localized)"="Packed Library:Get Non Exported Paths"}, "Method Flags"={"IsDeprecated"=FALSE, "IsPrivate"=TRUE, "IsScripting"=FALSE, "IsNotInRun-Time"=TRUE}, "Divider"=FALSE}, {"Class Info"={"Unique ID string"="80", "Parent ID string"="74", "Class Name (unlocalized)"="Library", "Class Name (localized)"="Library"}, "Method Info"={"Unique ID string"="4d10e425", "Data name"="NI Sec.Set ACL", "Short name (localized)"="NI Sec.Set ACL", "Long name (localized)"="NI Security:Set Access Control List"}, "Method Flags"={"IsDeprecated"=FALSE, "IsPrivate"=TRUE, "IsScripting"=TRUE, "IsNotInRun-Time"=FALSE}, "Divider"=FALSE}, {"Class Info"={"Unique ID string"="80", "Parent ID string"="74", "Class Name (unlocalized)"="Library", "Class Name (localized)"="Library"}, "Method Info"={"Unique ID string"="4d10e426", "Data name"="SaveBinary", "Short name (localized)"="SaveBinary", "Long name (localized)"="SaveBinary"}, "Method Flags"={"IsDeprecated"=FALSE, "IsPrivate"=TRUE, "IsScripting"=FALSE, "IsNotInRun-Time"=FALSE}, "Divider"=FALSE}, {"Class Info"={"Unique ID string"="80", "Parent ID string"="74", "Class Name (unlocalized)"="Library", "Class Name (localized)"="Library"}, "Method Info"={"Unique ID string"="4d10e427", "Data name"="Save a Shifted Copy", "Short name (localized)"="Save a Shifted Copy", "Long name (localized)"="Save:Shifted Copy"}, "Method Flags"={"IsDeprecated"=FALSE, "IsPrivate"=TRUE, "IsScripting"=FALSE, "IsNotInRun-Time"=TRUE}, "Divider"=FALSE}, {"Class Info"={"Unique ID string"="81", "Parent ID string"="", "Class Name (unlocalized)"="Variable", "Class Name (localized)"="Variable"}, "Method Info"={"Unique ID string"="4f483800", "Data name"="DisconnectFromTypedefs", "Short name (localized)"="DisconnectFromTypedefs", "Long name (localized)"="Disconnect From Typedefs"}, "Method Flags"={"IsDeprecated"=FALSE, "IsPrivate"=FALSE, 
